vi "ReferenceCursorORTForceCurves.vi"(8 "error in":errorcluster) -> (0 "error out":errorcluster, 2 "vi reference":refnum<vi>, 3 "Graphreference":refnum<vi>)   [LabVIEW 2016]
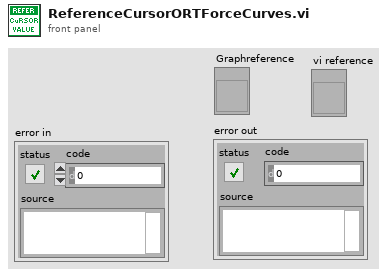
[diagram p1: front panel]
types:
  T1 = enum32{"Bad", "Idle", "Run top level", "Running"}
  T2 = enum32{"Invalid", "Standard", "Closed", "Hidden", "Minimized", "Maximized"}
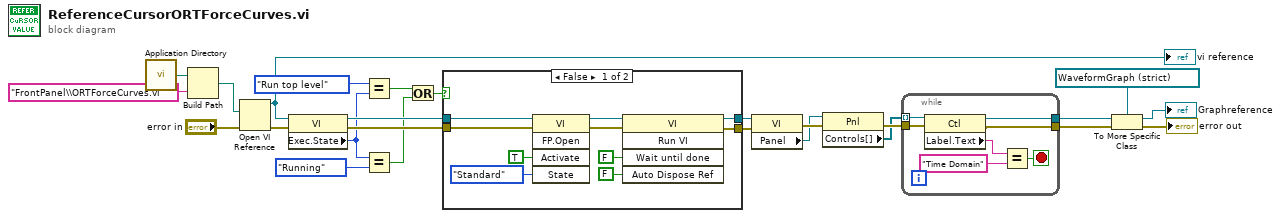
[diagram p0: block diagram]
diagram:
  n1 = call <vilib>:"Application Directory.vi"() -> ("Application Directory"=w19:path)
  n2 = Build Path(base path=w19, name or relative path="FrontPanel\\ORTForceCurves.vi") -> (appended path=w18:path)
  n3 = Open VI Reference(vi path=w18, error in (no error)="error in") -> (vi reference=w4:refnum<vi>, error out=w5:errorcluster)  [unwired: 4 in]
  "vi reference" <- w4
  n4 = property class="VI"(reference=w4, error in=w5) -> (reference out=w15:refnum<vi>, error out=w14:errorcluster, "Exec.State"=w9:T1)
  n5 = Equal?(x=T1."Run top level" ("Execution:State"), y=w9) -> (x = y?=w11:bool)
  n6 = Equal?(x=w9, y=T1."Running" ("Execution:State")) -> (x = y?=w10:bool)
  n7 = Or(x=w11, y=w10) -> (x .or. y?=w8:bool)
  n8 = case shown="False" w8 {
    tunnel: [w30 w36] -> w7
    tunnel: [w29 w37] -> w6
    tunnel: w15 -> [w27 w37]
    tunnel: w14 -> [w26 w36]
    frame False {
      n9 = invoke class="VI" method="FP.Open"(reference=w27, error in=w26, "Activate"=TRUE ("Activate?"), "State"=T2."Standard") -> (reference out=w32:refnum<vi>, error out=w31:errorcluster)  [unwired: 1 in, 3 out]
      n10 = invoke class="VI" method="Run VI"(reference=w32, error in=w31, "Wait until done"=FALSE ("Wait Until Done"), "Auto Dispose Ref"=FALSE ("Auto Dispose Reference")) -> (reference out=w29:refnum<vi>, error out=w30:errorcluster)  [unwired: 1 in, 3 out]
    }
    frame True {
    }
  }
  n11 = property class="VI"(reference=w6, error in=w7) -> (error out=w24:errorcluster, "Panel"=w17:refnum<vi>)  [unwired: 1 out]
  n12 = property class="Pnl"(reference=w17, error in=w24) -> (error out=w25:errorcluster, "Controls[]"=w21:refnum<vi>[])  [unwired: 1 out]
  n13 = while {
    tunnel: w21 -> [w44] mode=indexing
    tunnel: [w42] -> w22
    tunnel: [w41] -> w23
    tunnel: w25 -> [w40]
    stop <- w39 stop-if-true
    n14 = property class="Ctl"(reference=w44, error in=w40) -> (reference out=w42:refnum<vi>, error out=w41:errorcluster, "Label.Text"=w38:string)
    n15 = Equal?(x=w38, y="Time Domain") -> (x = y?=w39:bool)
  }
  n16 = To More Specific Class(target class=refnum<vi> refnum ("interactionTimeDomain"), reference=w22, error in=w23) -> (specific class reference=→"Graphreference":refnum<vi>, error out=→"error out":errorcluster)
